vi "record_fiberphotometry_animalbehavior.vi"() -> ()   [LabVIEW 2020]
uses:
  <vilib>/vision/driver/IMAQdx.llb/IMAQdx Buffer Number Mode.ctl
  <vilib>/userDefined/High Color/IMAQdx.ctl
  <userlib>/AndorSDK3/Data/GetPixelData16.vi
  <vilib>/vision/driver/NI_Vision_Acquisition_Software.lvlib
panel:
  in  "Aquisition interval (s)":dbl
  in  "Camera Exposure(s)":dbl
  in  "AOI Top":i64
  in  "AOI Left":i64
  in  "moviefile name":string
  in  "Behavior Data Path":path
  in  "Measurement period (min)":dbl
  in  "Sampling rate (Hz)":i32=5
  in  "error constant":errorcluster
  in  "USB camera":T1
  in  "stop 2":bool
  in  "Buffer Number Mode (Next)":T2
  out "Image":T3(plugin-control)
  in  "405 nm power(%)":i32
  in  "470 nm power (%)":i32
  in  "Imaging Data Path":path
  in  "Binning":string
  in  "Apply Settings":bool
  in  "stop":bool
  in  "count":i32
  in  "image pointers":u64[](array[numeric])
  in  "imageNo":i32 caption="Displayed image" min=0 max=75
  in  "NumImages":i32=10
  in  "Centre AOI":bool
  in  "AOI Width":i64
  in  "AOI Height":i64
  out "Ready":bool
  in  "Run":bool
  in  "error":errorcluster
  out "Pixel Encoding":string
  out "Intensity Graph":u16[][](graph)
  out "AOIStride":i64
  in  "PreAmp Gain Control":string(combo)
  out "PixelData":u16[](array[numeric])
  out "ByteData":u8[](array[numeric])
  out "ImageSizeBytes":i64
  out "Handle":i32
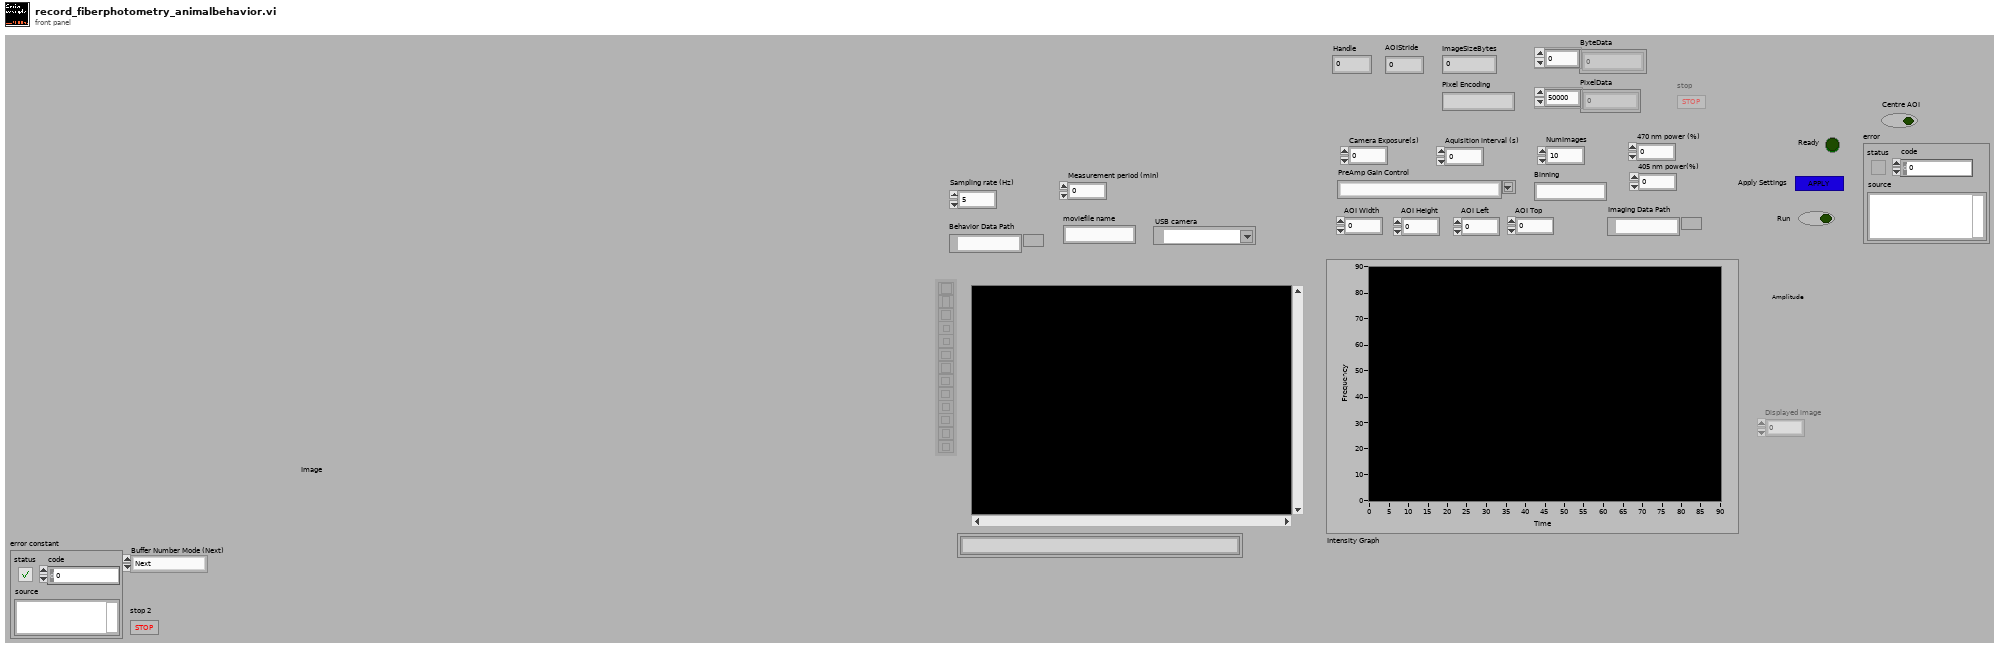
[diagram p1: front panel]
types:
  T1 = typedef "IMAQdx.ctl" = refnum<k21>
  T2 = typedef "NI_Vision_Acquisition_Software.lvlib/IMAQdx Buffer Number Mode.ctl" = enum32{"Next", "Last", "Buffer Number", "Every", "Last New"}
  T3 = typedef "IMAQ Image.ctl" = refnum<image>
  T4 = enum8{"Enabled", "Disabled", "Disabled and Grayed Out"}
  T5 = typedef "Image Type" = u32
  T6 = typedef "AviRefnum.ctl" = refnum<k1>
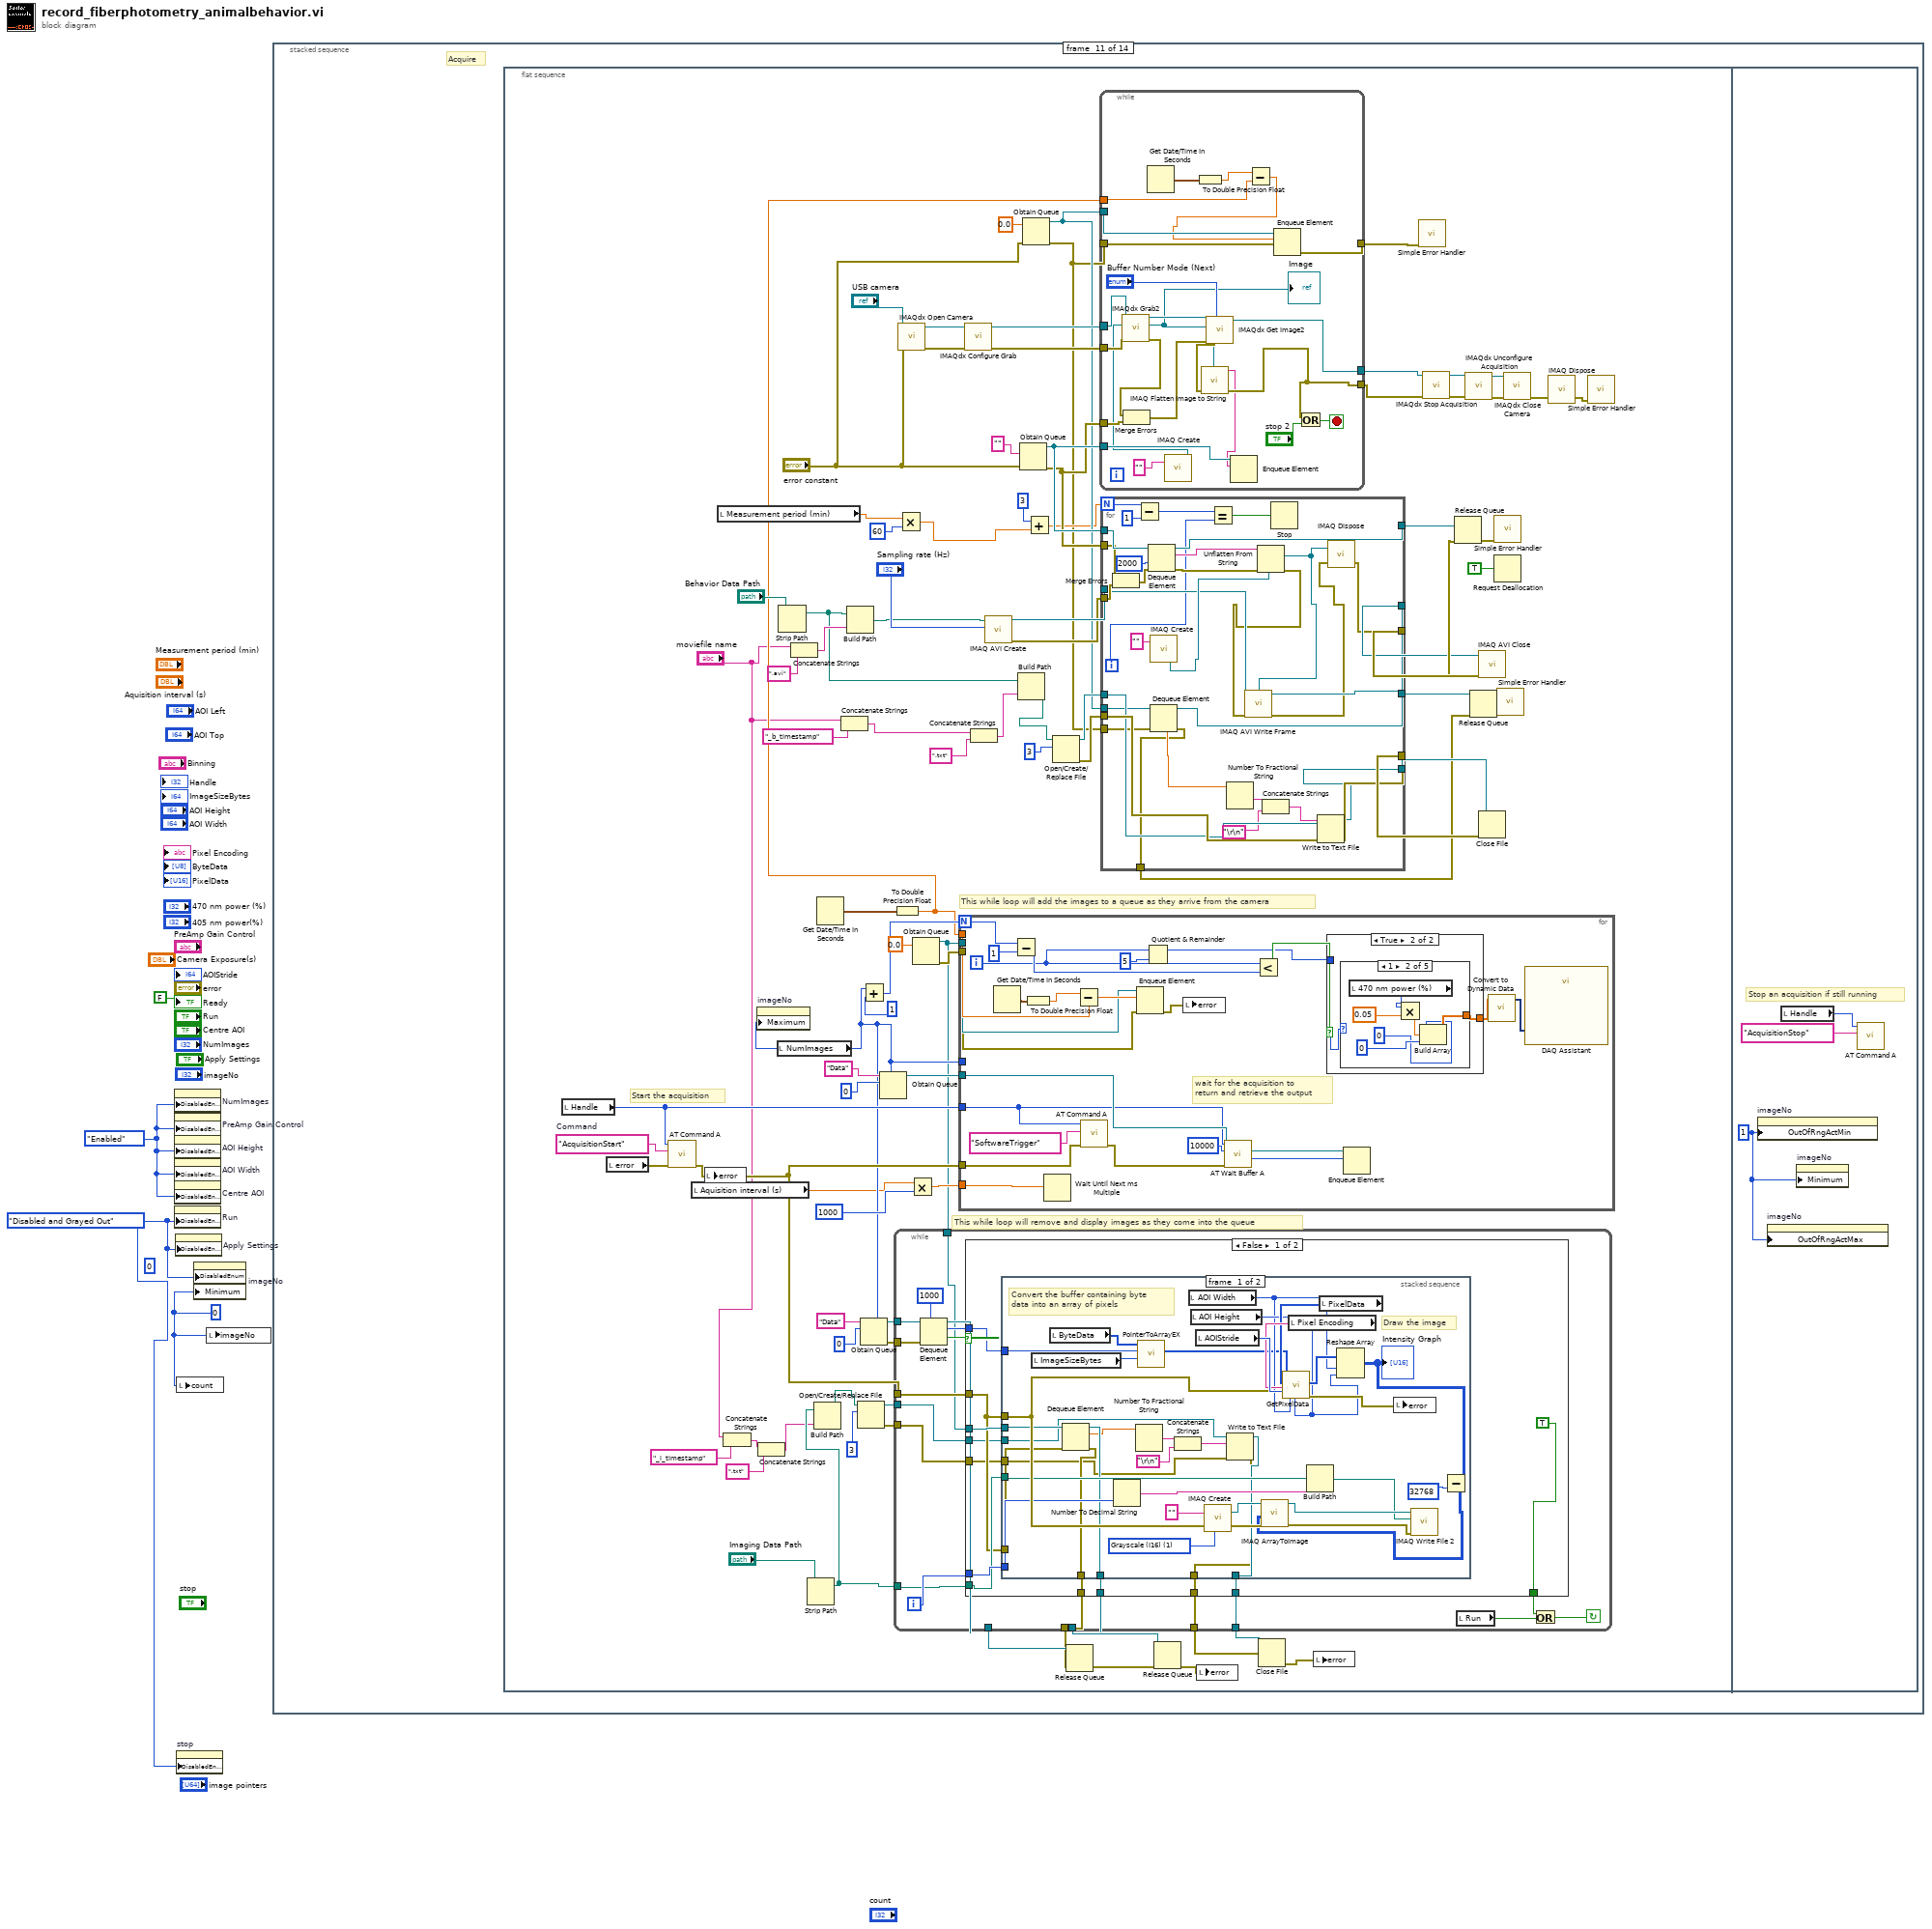
[diagram p0: block diagram]
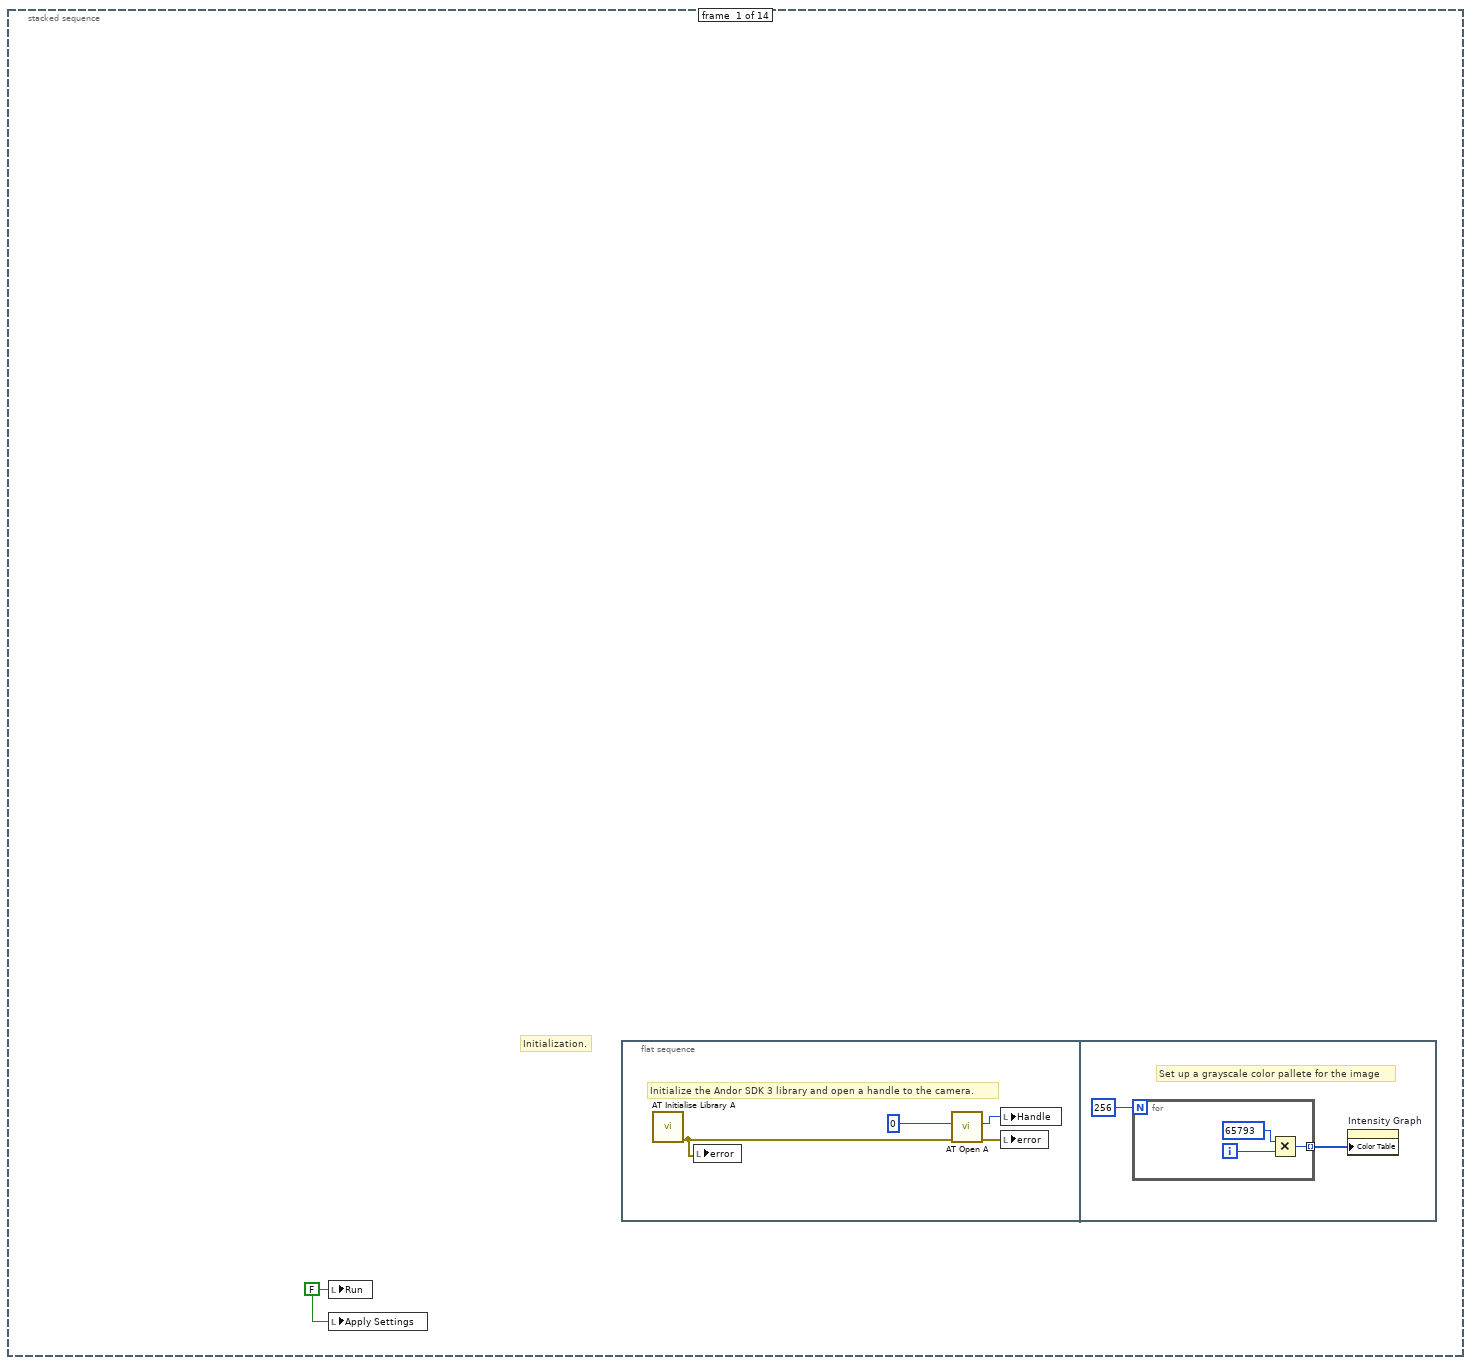
[diagram p2: hidden frame]
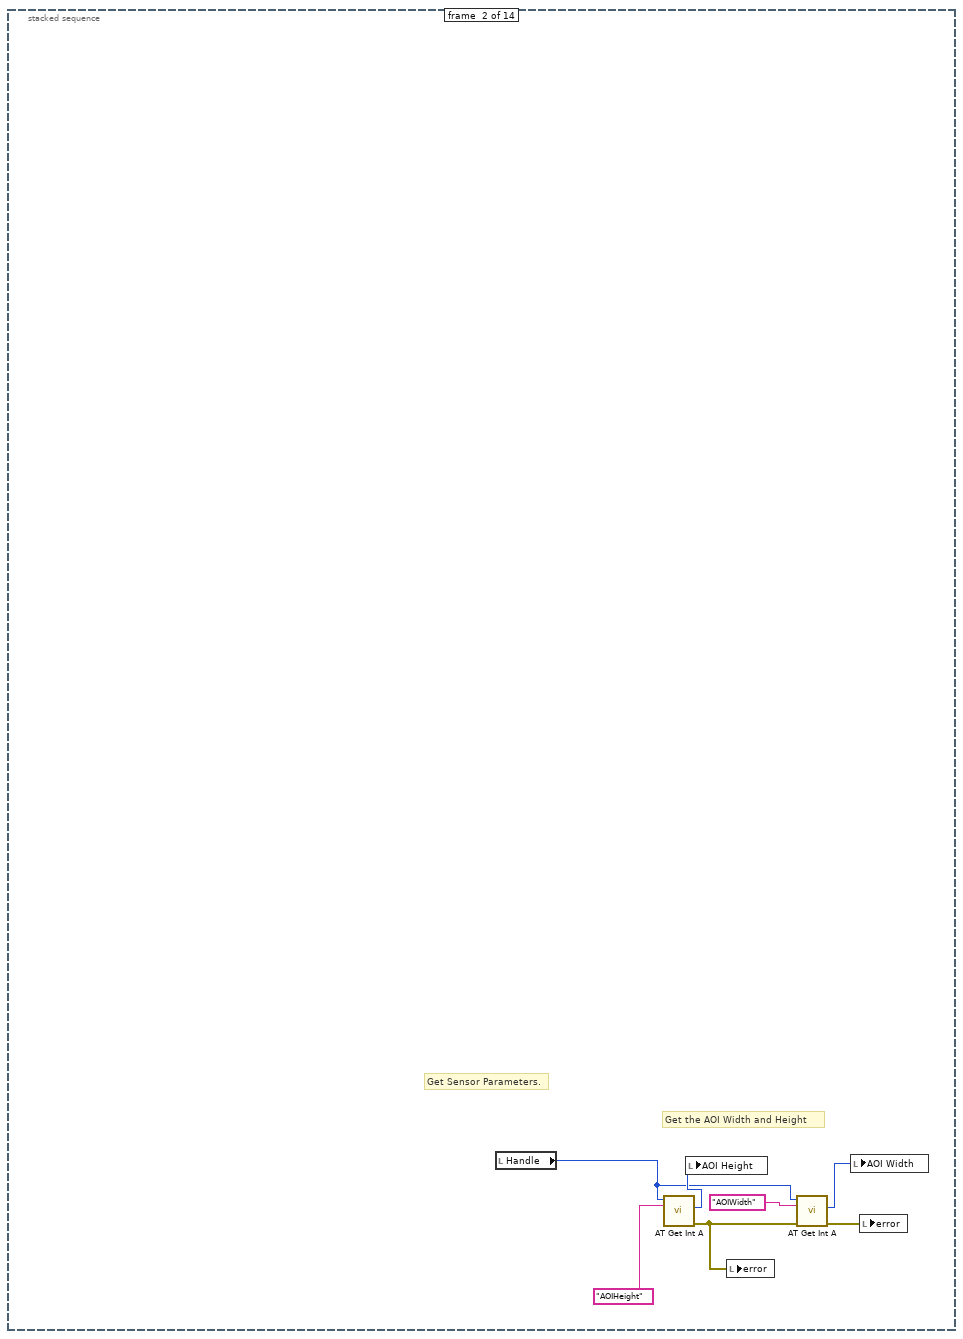
[diagram p3: hidden frame]
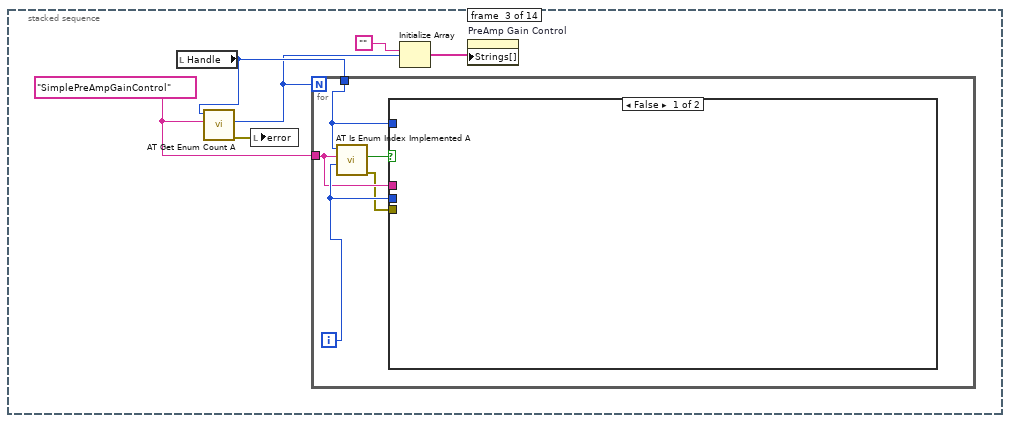
[diagram p4: hidden frame]
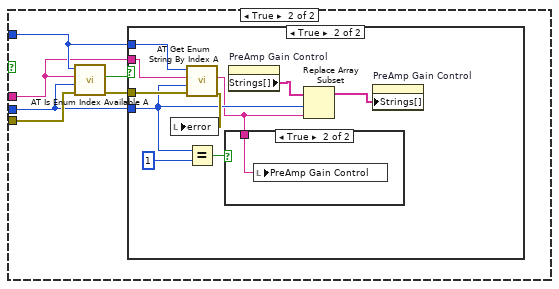
[diagram p5: hidden frame]
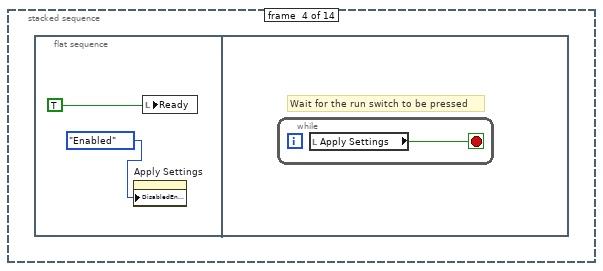
[diagram p8: hidden frame]
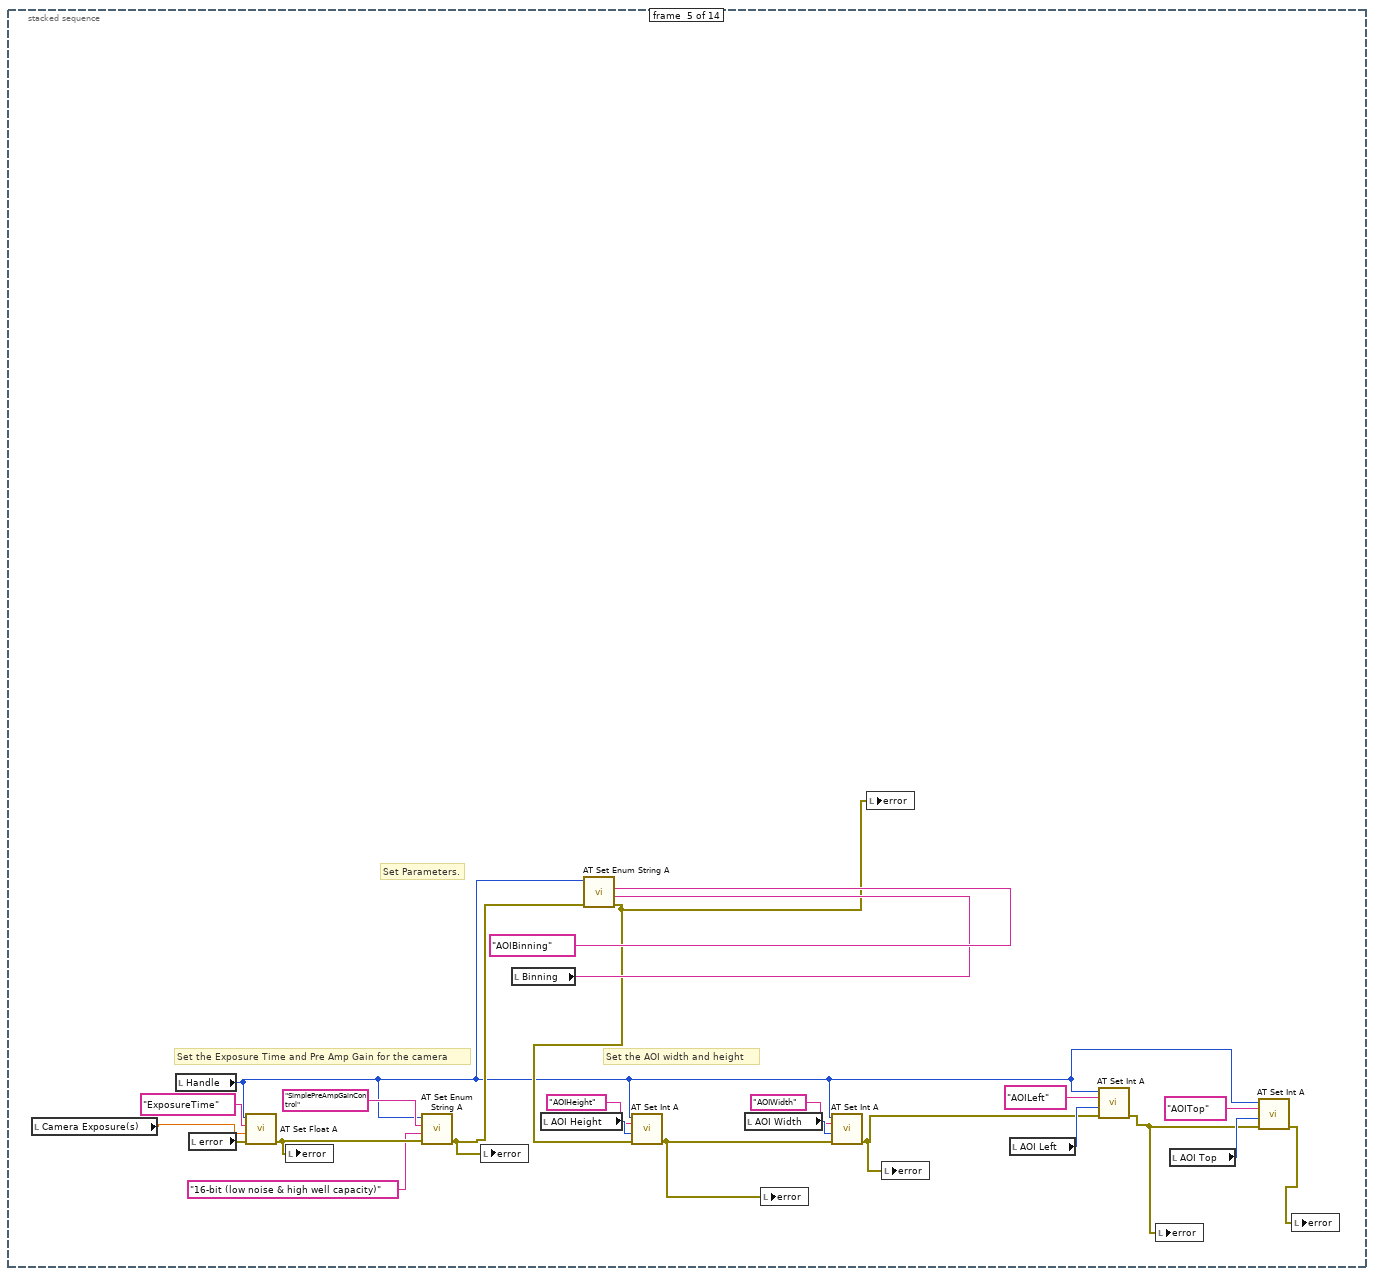
[diagram p9: hidden frame]
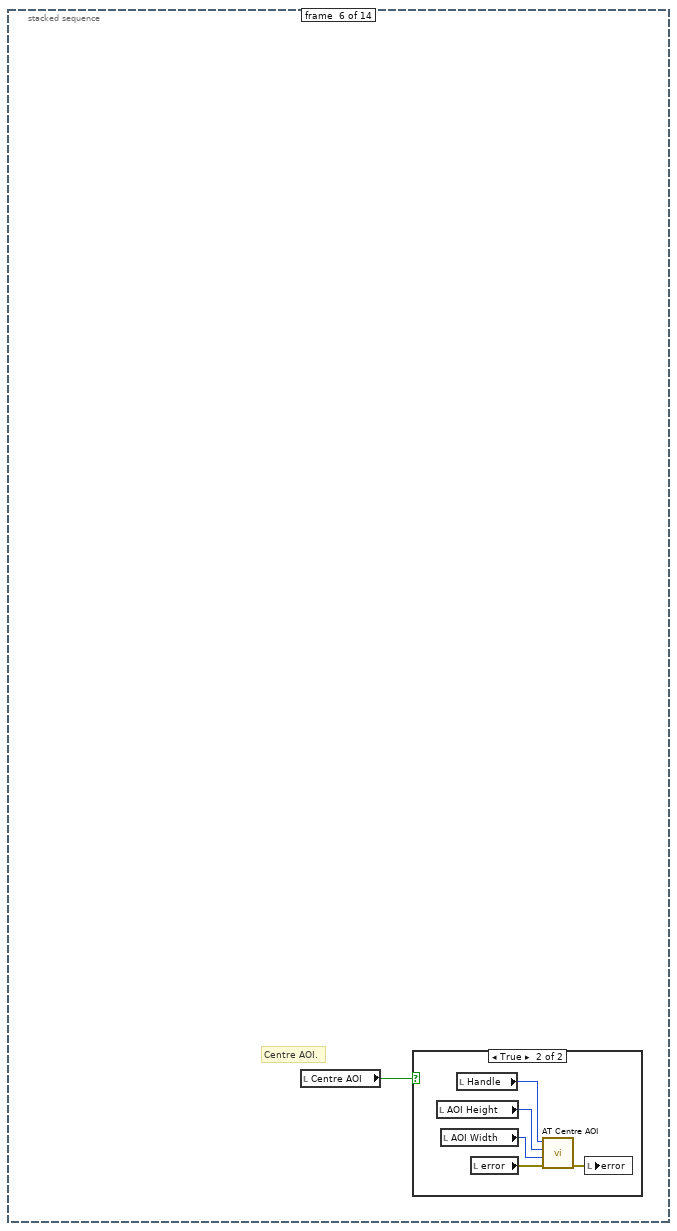
[diagram p10: hidden frame]
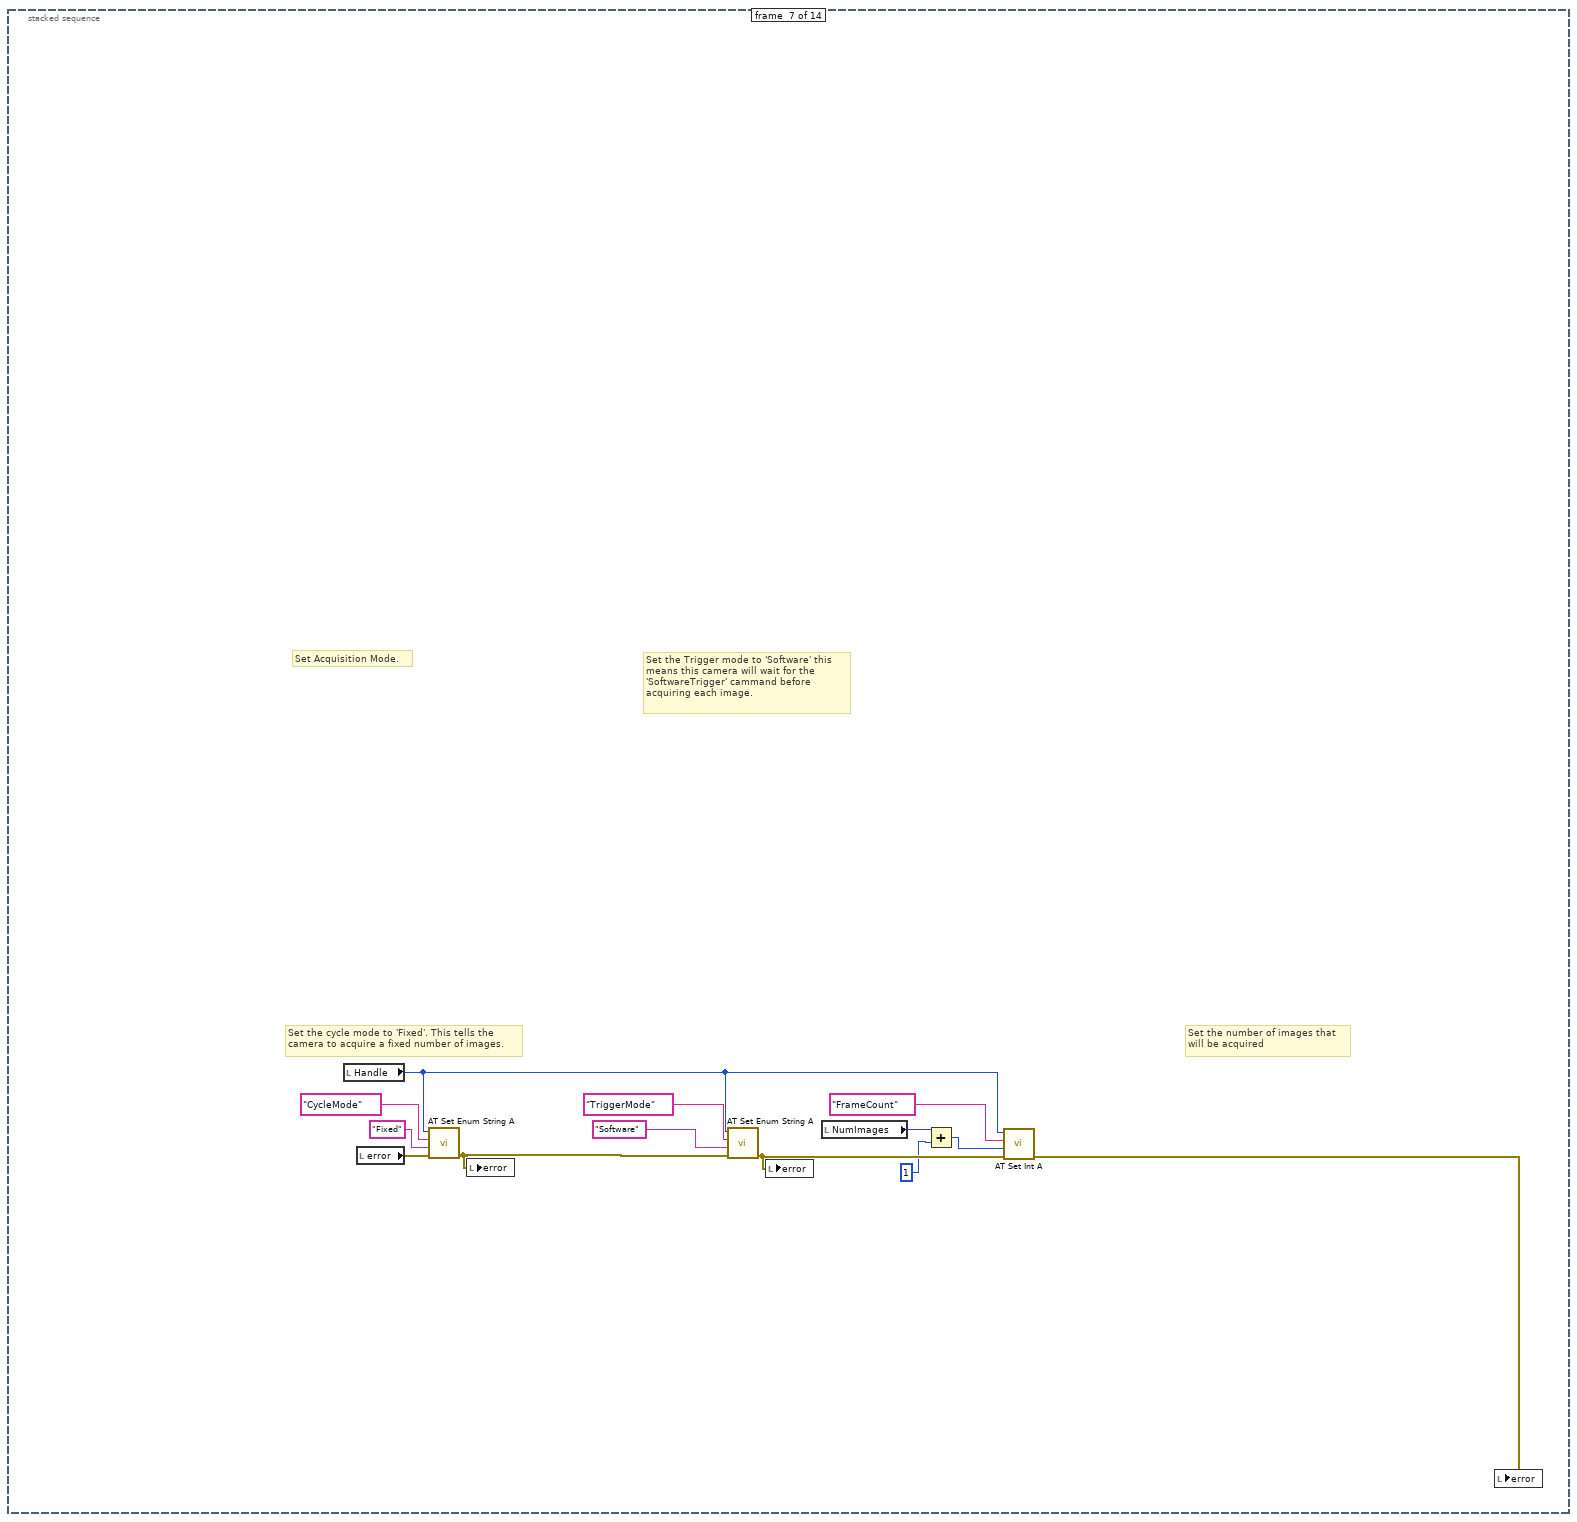
[diagram p12: hidden frame]
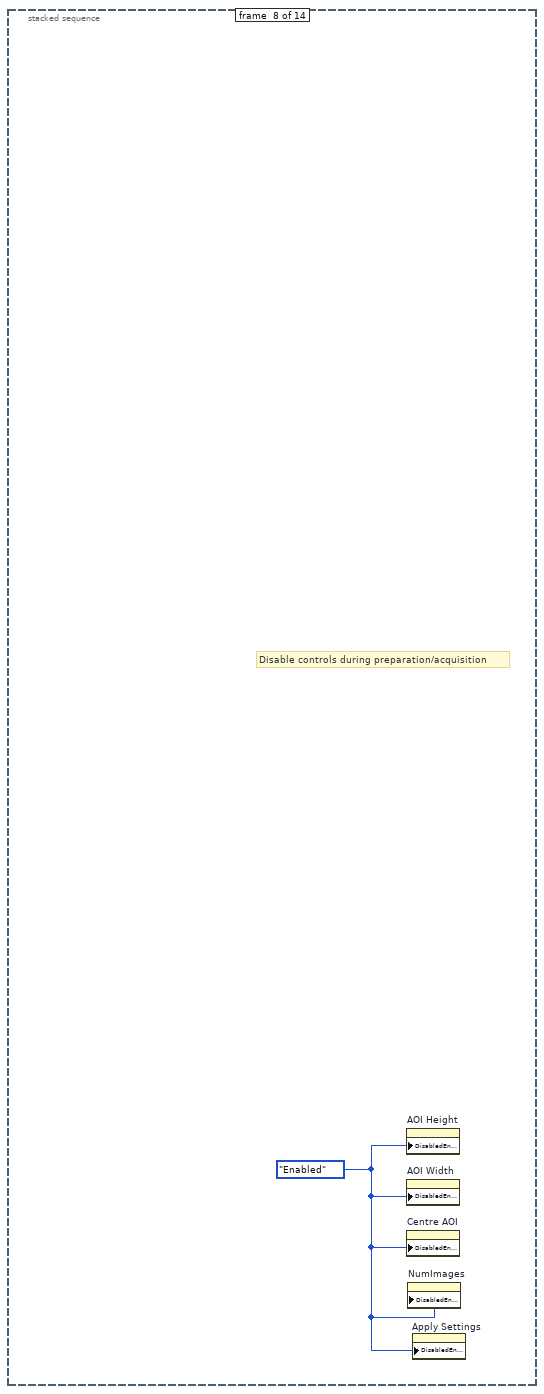
[diagram p13: hidden frame]
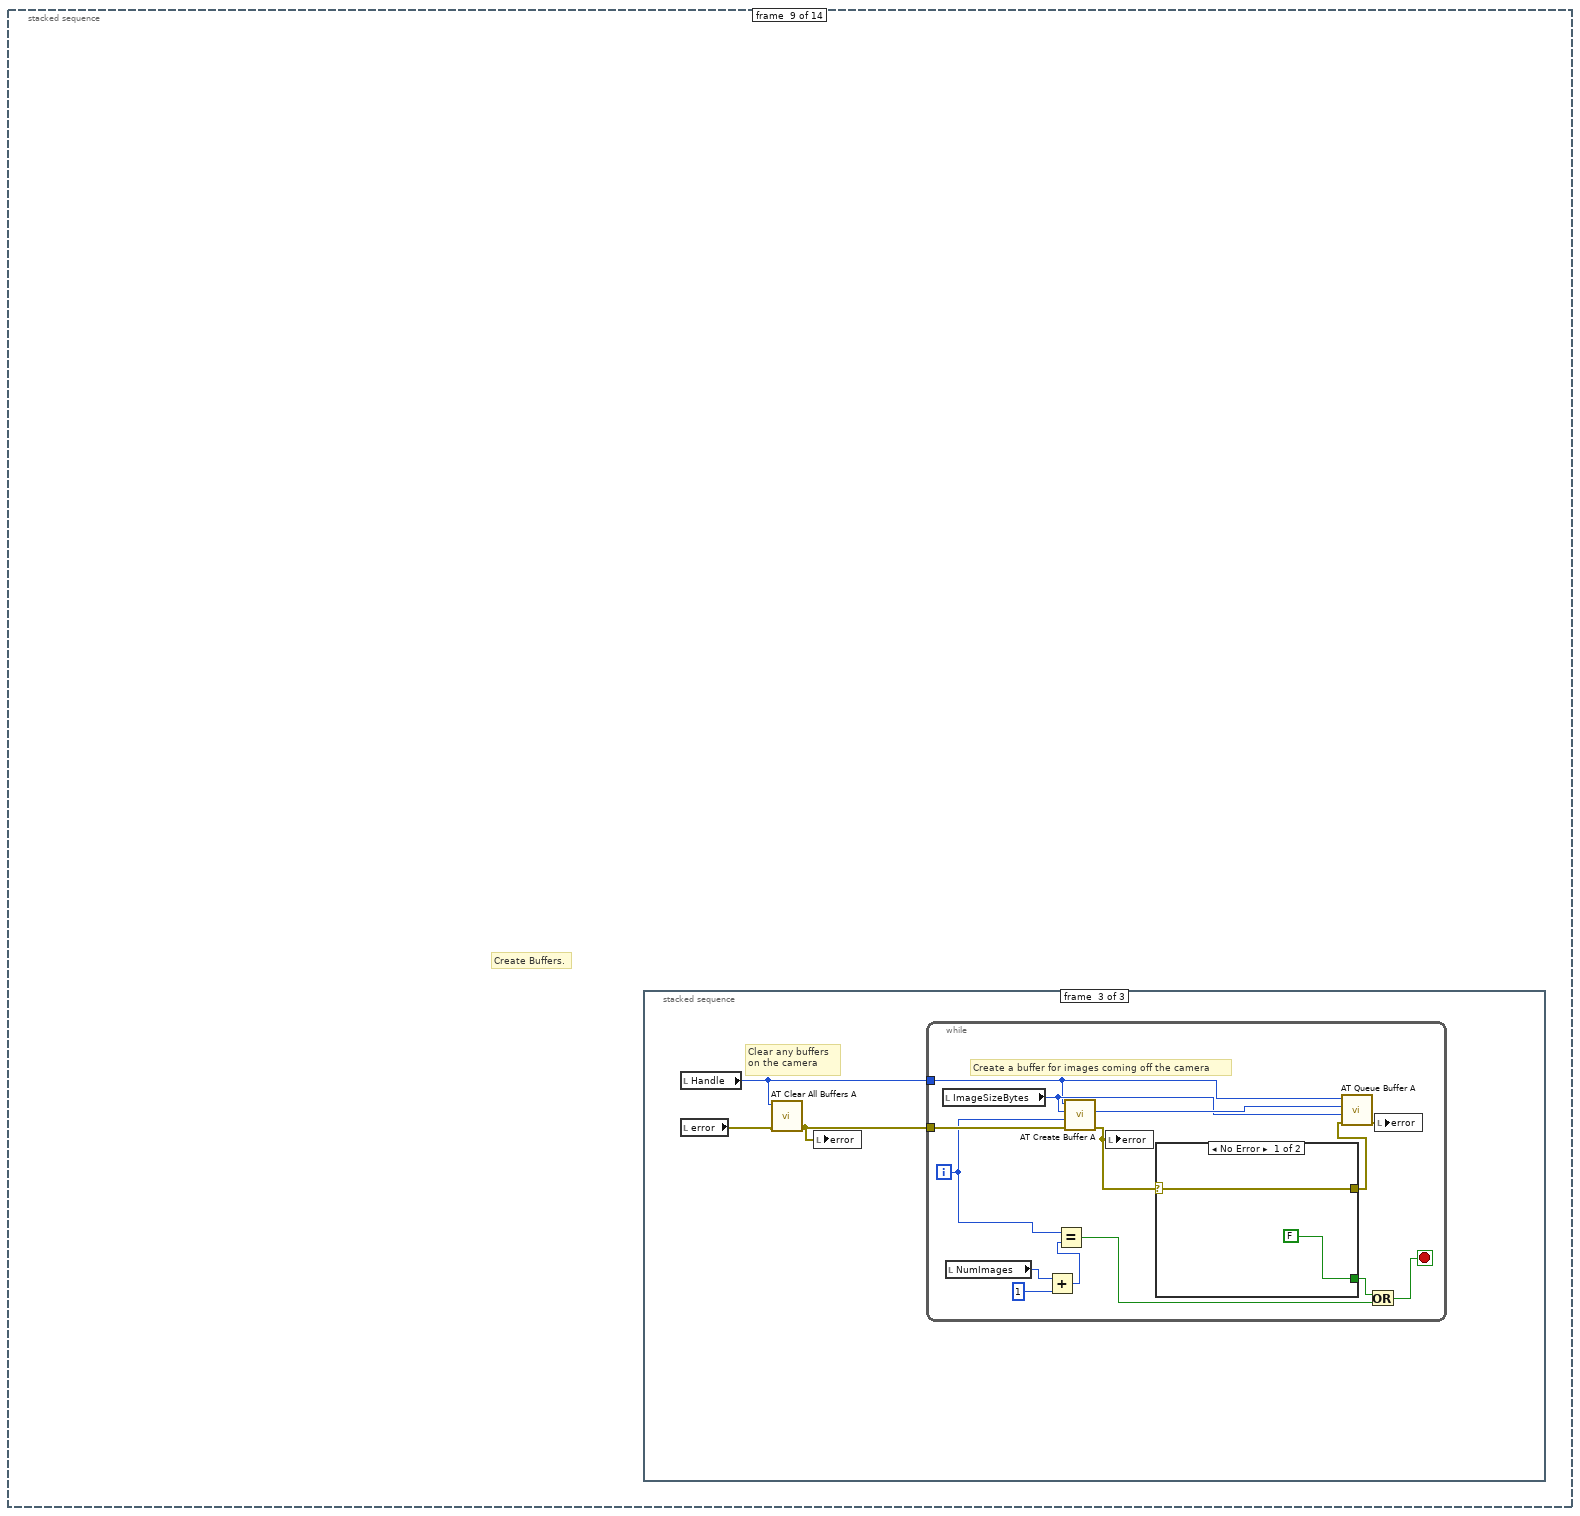
[diagram p14: hidden frame]
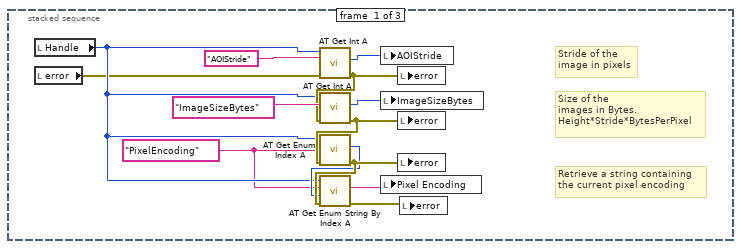
[diagram p15: hidden frame]
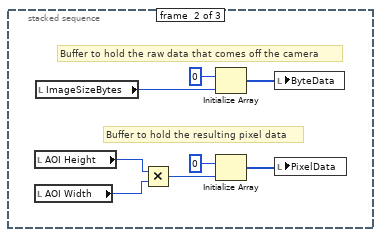
[diagram p16: hidden frame]
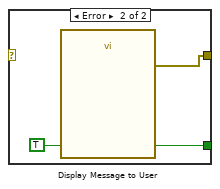
[diagram p17: hidden frame]
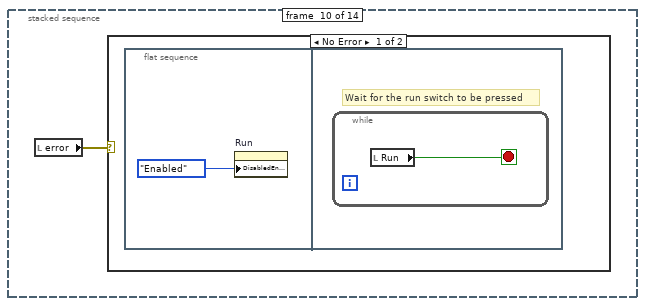
[diagram p18: hidden frame]
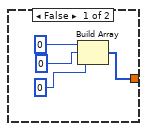
[diagram p20: hidden frame]
diagram:
  w2 = 0 ("Data Entry Limits:Minimum")
  (unwired) 0 ("Image")
  w1 = T4."Disabled and Grayed Out" ("Disabled")
  w3 = T4."Enabled" ("Disabled")
  n1 = property on="NumImages" class="DigNum (strict)"("DisabledEnum"=w3) -> ()  [unwired: 2 in, 2 out]
  n2 = property on="PreAmp Gain Control" class="CmbBox"("DisabledEnum"=w3) -> ()  [unwired: 2 in, 2 out]
  n3 = property on="AOI Height" class="DigNum (strict)"("DisabledEnum"=w3) -> ()  [unwired: 2 in, 2 out]
  n4 = property on="AOI Width" class="DigNum (strict)"("DisabledEnum"=w3) -> ()  [unwired: 2 in, 2 out]
  n5 = property on="Centre AOI" class="Bool (strict)"("DisabledEnum"=w3) -> ()  [unwired: 2 in, 2 out]
  n6 = property on="Run" class="Bool (strict)"("DisabledEnum"=w1) -> ()  [unwired: 2 in, 2 out]
  n7 = property on="Apply Settings" class="Bool (strict)"("DisabledEnum"=w1) -> ()  [unwired: 2 in, 2 out]
  n8 = local write "count"(w2) -> ()
  n9 = property on="stop" class="Bool (strict)"("DisabledEnum"=w1) -> ()  [unwired: 2 in, 2 out]
  n10 = property on="imageNo" class="DigNum (strict)"("DisabledEnum"=w1, "Minimum"=w2) -> ()  [unwired: 2 in, 2 out]
  n11 = local write "imageNo"(w2) -> ()
  n12 = stacked-sequence {
    frame #0 {
      w5 = FALSE ("Run")
      # "Initialization."
      n13 = local write "Run"(w5) -> ()
      n14 = local write "Apply Settings"(w5) -> ()
      n15 = flat-sequence {
        frame #0 {
          # "Initialize the Andor SDK 3 library and open a handle to the camera."
          n16 = call <userlib>:"AT Initialise Library A.vi"() -> ("error out"=w7:errorcluster)  [unwired: 10 in, 1 out]
          n17 = local write "error"(w7) -> ()
          n18 = call <userlib>:"AT Open A.vi"("error in (no error)"=w7, "CameraIndex"=0) -> ("error out"=w6:errorcluster, "Handle"=w8:i32)  [unwired: 7 in, 1 out]
          n19 = local write "Handle"(w8) -> ()
          n20 = local write "error"(w6) -> ()
        }
        frame #1 {
          # "Set up a grayscale color pallete for the image"
          n21 = for {
            N: 256 -> [_]
            tunnel: [w13] -> w10 mode=indexing
            i -> [w14]
            n22 = Multiply(x=65793, y=w14) -> (x*y=w13:i32)
          }
          n23 = property on="Intensity Graph" class="IntGraph (strict)"("Color Table"=w10) -> ()  [unwired: 2 in, 2 out]
        }
      }
    }
    frame #1 {
      # "Get the AOI Width and Height"
      # "Get Sensor Parameters."
      n24 = local read "Handle"() -> (w15:i32)
      n25 = call <userlib>:"AT Get Int A.vi"("Feature"="AOIHeight" ("Integer feature 2"), "Handle"=w15) -> ("error out"=w18:errorcluster, "Value"=w16:i64)  [unwired: 7 in, 1 out]
      n26 = local write "AOI Height"(w16) -> ()
      n27 = local write "error"(w18) -> ()
      n28 = call <userlib>:"AT Get Int A.vi"("error in (no error)"=w18, "Feature"="AOIWidth" ("Integer feature"), "Handle"=w15) -> ("error out"=w21:errorcluster, "Value"=w17:i64)  [unwired: 6 in, 1 out]
      n29 = local write "AOI Width"(w17) -> ()
      n30 = local write "error"(w21) -> ()
    }
    frame #2 {
      w22 = "SimplePreAmpGainControl" ("Enum feature")
      n31 = local read "Handle"() -> (w26:i32)
      n32 = call <userlib>:"AT Get Enum Count A.vi"("Feature"=w22, "Handle"=w26) -> ("error out"=w27:errorcluster, "Count"=w25:i32)  [unwired: 7 in, 1 out]
      n33 = local write "error"(w27) -> ()
      n34 = for {
        N: w25 -> [_]
        tunnel: w26 -> [w29]
        tunnel: w22 -> [w30]
        i -> [w31]
        n35 = call <userlib>:"AT Is Enum Index Implemented A.vi"("Index"=w31, "Feature"=w30, "Handle"=w29) -> ("error out"=w28:errorcluster, "Implemented"=w32:bool)  [unwired: 6 in, 1 out]
        n36 = case shown="False" w32 {
          tunnel: w31 -> [_ w34]
          tunnel: w30 -> [_ w35]
          tunnel: w29 -> [_ w36]
          tunnel: w28 -> [_ w38]
          frame False {
          }
          frame True {
            n37 = call <userlib>:"AT Is Enum Index Available A.vi"("error in (no error)"=w38, "Index"=w34, "Feature"=w35, "Handle"=w36) -> ("error out"=w33:errorcluster, "Available"=w37:bool)  [unwired: 5 in, 1 out]
            n38 = case shown="True" w37 {
              tunnel: w36 -> [_ w48]
              tunnel: w35 -> [_ w47]
              tunnel: w34 -> [_ w44]
              tunnel: w33 -> [_ w46]
              frame False {
              }
              frame True {
                n39 = call <userlib>:"AT Get Enum String By Index A.vi"("error in (no error)"=w46, "Index"=w44, "Feature"=w47, "Handle"=w48) -> ("error out"=w45:errorcluster, "String"=w41:string)  [unwired: 5 in, 1 out]
                n40 = local write "error"(w45) -> ()
                n41 = Equal?(x=w44, y=1) -> (x = y?=w42:bool)
                n42 = case shown="True" w42 {
                  tunnel: w41 -> [_ w49]
                  frame False {
                  }
                  frame True {
                    n43 = local write "PreAmp Gain Control"(w49) -> ()
                  }
                }
                n44 = property on="PreAmp Gain Control" class="CmbBox"() -> ("Strings[]"=w40:string[])  [unwired: 2 in, 2 out]
                n45 = Replace Array Subset(array=w40, new element=w41, index=w44) -> (w39:string[])
                n46 = property on="PreAmp Gain Control" class="CmbBox"("Strings[]"=w39) -> ()  [unwired: 2 in, 2 out]
              }
            }
          }
        }
      }
      n47 = Initialize Array("", w25) -> (w23:string[])
      n48 = property on="PreAmp Gain Control" class="CmbBox"("Strings[]"=w23) -> ()  [unwired: 2 in, 2 out]
    }
    frame #3 {
      n49 = flat-sequence {
        frame #0 {
          n50 = property on="Apply Settings" class="Bool (strict)"("DisabledEnum"=T4."Enabled" ("Disabled")) -> ()  [unwired: 2 in, 2 out]
          n51 = local write "Ready"(TRUE ("Ready")) -> ()
        }
        frame #1 {
          # "Wait for the run switch to be pressed"
          n52 = while {
            stop <- w52 stop-if-true
            n53 = local read "Apply Settings"() -> (w52:bool)
          }
        }
      }
    }
    frame #4 {
      # "Set the AOI width and height"
      # "Set the Exposure Time and Pre Amp Gain for the camera"
      # "Set Parameters."
      n54 = local read "Camera Exposure(s)"() -> (w53:dbl)
      n55 = local read "Handle"() -> (w54:i32)
      n56 = local read "error"() -> (w73:errorcluster)
      n57 = call <userlib>:"AT Set Float A.vi"("error in (no error)"=w73, "Value"=w53, "Feature"="ExposureTime" ("ExposureTime"), "Hndl"=w54) -> ("error out"=w75:errorcluster)  [unwired: 6 in, 1 out]
      n58 = local write "error"(w75) -> ()
      n59 = call <userlib>:"AT Set Enum String A.vi"("error in (no error)"=w75, "String"="16-bit (low noise & high well capacity)", "Feature"="SimplePreAmpGainControl" ("Enum feature"), "Handle"=w54) -> ("error out"=w64:errorcluster)  [unwired: 6 in, 1 out]
      n60 = local write "error"(w64) -> ()
      n61 = local read "Binning"() -> (w65:string)
      n62 = local read "AOI Height"() -> (w71:i64)
      n63 = call <userlib>:"AT Set Enum String A.vi"("error in (no error)"=w64, "String"=w65, "Feature"="AOIBinning" ("Enum feature"), "Handle"=w54) -> ("error out"=w63:errorcluster)  [unwired: 6 in, 1 out]
      n64 = call <userlib>:"AT Set Int A.vi"("error in (no error)"=w63, "Value"=w71, "Feature"="AOIHeight" ("Integer feature"), "Handle"=w54) -> ("error out"=w72:errorcluster)  [unwired: 6 in, 1 out]
      n65 = local read "AOI Width"() -> (w70:i64)
      n66 = local write "error"(w72) -> ()
      n67 = call <userlib>:"AT Set Int A.vi"("error in (no error)"=w72, "Value"=w70, "Feature"="AOIWidth" ("Integer feature 2"), "Handle"=w54) -> ("error out"=w55:errorcluster)  [unwired: 6 in, 1 out]
      n68 = local write "error"(w63) -> ()
      n69 = local write "error"(w55) -> ()
      n70 = local read "AOI Left"() -> (w61:i64)
      n71 = call <userlib>:"AT Set Int A.vi"("error in (no error)"=w55, "Value"=w61, "Feature"="AOILeft" ("Integer feature 2"), "Handle"=w54) -> ("error out"=w56:errorcluster)  [unwired: 6 in, 1 out]
      n72 = local write "error"(w56) -> ()
      n73 = local read "AOI Top"() -> (w59:i64)
      n74 = call <userlib>:"AT Set Int A.vi"("error in (no error)"=w56, "Value"=w59, "Feature"="AOITop" ("Integer feature 2"), "Handle"=w54) -> ("error out"=w57:errorcluster)  [unwired: 6 in, 1 out]
      n75 = local write "error"(w57) -> ()
    }
    frame #5 {
      # "Centre AOI."
      n76 = local read "Centre AOI"() -> (w76:bool)
      n77 = case shown="True" w76 {
        frame False {
        }
        frame True {
          n78 = local read "AOI Height"() -> (w78:i64)
          n79 = local read "AOI Width"() -> (w79:i64)
          n80 = local read "Handle"() -> (w77:i32)
          n81 = local read "error"() -> (w80:errorcluster)
          n82 = call <userlib>:"AT Centre AOI.vi"("error in (no error)"=w80, "AOI Width"=w79, "AOI Height"=w78, "Handle"=w77) -> ("error out"=w81:errorcluster)  [unwired: 7 in]
          n83 = local write "error"(w81) -> ()
        }
      }
    }
    frame #6 {
      # "Set the number of images that \nwill be acquired"
      # "Set the Trigger mode to 'Software' this \nmeans this camera will wait for the \n'SoftwareTrigger' cammand before \nacquiring each image."
      # "Set the cycle mode to 'Fixed'. This tells the \ncamera to acquire a fixed number of images."
      # "Set Acquisition Mode."
      n84 = local read "Handle"() -> (w88:i32)
      n85 = local read "error"() -> (w93:errorcluster)
      n86 = call <userlib>:"AT Set Enum String A.vi"("error in (no error)"=w93, "String"="Fixed", "Feature"="CycleMode" ("Enum feature"), "Handle"=w88) -> ("error out"=w92:errorcluster)  [unwired: 6 in, 1 out]
      n87 = local write "error"(w92) -> ()
      n88 = call <userlib>:"AT Set Enum String A.vi"("error in (no error)"=w92, "String"="Software", "Feature"="TriggerMode" ("Enum feature"), "Handle"=w88) -> ("error out"=w90:errorcluster)  [unwired: 6 in, 1 out]
      n89 = local write "error"(w90) -> ()
      n90 = local read "NumImages"() -> (w84:i32)
      n91 = Add(x=w84, y=1) -> (x+y=w82:i32)
      n92 = call <userlib>:"AT Set Int A.vi"("error in (no error)"=w90, "Value"=w82, "Feature"="FrameCount" ("Integer feature 2"), "Handle"=w88) -> ("error out"=w85:errorcluster)  [unwired: 6 in, 1 out]
      n93 = local write "error"(w85) -> ()
    }
    frame #7 {
      w95 = T4."Enabled" ("Disabled")
      # "Disable controls during preparation/acquisition"
      n94 = property on="AOI Height" class="DigNum (strict)"("DisabledEnum"=w95) -> ()  [unwired: 2 in, 2 out]
      n95 = property on="AOI Width" class="DigNum (strict)"("DisabledEnum"=w95) -> ()  [unwired: 2 in, 2 out]
      n96 = property on="Centre AOI" class="Bool (strict)"("DisabledEnum"=w95) -> ()  [unwired: 2 in, 2 out]
      n97 = property on="NumImages" class="DigNum (strict)"("DisabledEnum"=w95) -> ()  [unwired: 2 in, 2 out]
      n98 = property on="Apply Settings" class="Bool (strict)"("DisabledEnum"=w95) -> ()  [unwired: 2 in, 2 out]
    }
    frame #8 {
      # "Create Buffers."
      n99 = stacked-sequence {
        frame #0 {
          w96 = "PixelEncoding" ("Enum feature")
          # "Retrieve a string containing \nthe current pixel encoding"
          # "Stride of the\nimage in pixels"
          # "Size of the\nimages in Bytes.\nHeight*Stride*BytesPerPixel"
          n100 = local read "Handle"() -> (w98:i32)
          n101 = local read "error"() -> (w97:errorcluster)
          n102 = call <userlib>:"AT Get Int A.vi"("error in (no error)"=w97, "Feature"="AOIStride" ("Integer feature"), "Handle"=w98) -> ("error out"=w104:errorcluster, "Value"=w108:i64)  [unwired: 6 in, 1 out]
          n103 = call <userlib>:"AT Get Int A.vi"("error in (no error)"=w104, "Feature"="ImageSizeBytes" ("Integer feature"), "Handle"=w98) -> ("error out"=w103:errorcluster, "Value"=w107:i64)  [unwired: 6 in, 1 out]
          n104 = call <userlib>:"AT Get Enum Index A.vi"("error in (no error)"=w103, "Feature"=w96, "Handle"=w98) -> ("error out"=w102:errorcluster, "Value"=w101:i32)  [unwired: 6 in, 1 out]
          n105 = call <userlib>:"AT Get Enum String By Index A.vi"("error in (no error)"=w102, "Index"=w101, "Feature"=w96, "Handle"=w98) -> ("error out"=w99:errorcluster, "String"=w100:string)  [unwired: 5 in, 1 out]
          n106 = local write "AOIStride"(w108) -> ()
          n107 = local write "ImageSizeBytes"(w107) -> ()
          n108 = local write "Pixel Encoding"(w100) -> ()
          n109 = local write "error"(w104) -> ()
          n110 = local write "error"(w103) -> ()
          n111 = local write "error"(w102) -> ()
          n112 = local write "error"(w99) -> ()
        }
        frame #1 {
          # "Buffer to hold the resulting pixel data"
          # "Buffer to hold the raw data that comes off the camera"
          n113 = local read "AOI Height"() -> (w114:i64)
          n114 = local read "AOI Width"() -> (w115:i64)
          n115 = local read "ImageSizeBytes"() -> (w110:i64)
          n116 = Multiply(x=w114, y=w115) -> (x*y=w109:i64)
          n117 = Initialize Array(u8 0, w110) -> (w112:u8[])
          n118 = Initialize Array(i64 0, w109) -> (w113:i64[])
          n119 = local write "ByteData"(w112) -> ()
          n120 = local write "PixelData"(w113) -> ()
        }
        frame #2 {
          # "Clear any buffers \non the camera"
          n121 = local read "Handle"() -> (w117:i32)
          n122 = local read "error"() -> (w119:errorcluster)
          n123 = call <userlib>:"AT Clear All Buffers A.vi"("error in (no error)"=w119, "Handle"=w117) -> ("error out"=w118:errorcluster)  [unwired: 8 in, 1 out]
          n124 = local write "error"(w118) -> ()
          n125 = while {
            tunnel: w118 -> [w130]
            tunnel: w117 -> [w129]
            i -> [w126]
            stop <- w123 stop-if-true
            # "Create a buffer for images coming off the camera"
            n126 = local read "ImageSizeBytes"() -> (w132:i64)
            n127 = local read "NumImages"() -> (w122:i32)
            n128 = Add(x=w122, y=1) -> (x+y=w120:i32)
            n129 = Equal?(x=w126, y=w120) -> (x = y?=w124:bool)
            n130 = call <userlib>:"AT Create Buffer A.vi"("error in (no error)"=w130, "Buffer"=w126, "Size"=w132, "Handle"=w129) -> ("error out"=w128:errorcluster, "Buffer out"=w133:u64)  [unwired: 5 in, 1 out]
            n131 = local write "error"(w128) -> ()
            n132 = case shown="No Error" w128 {
              selector: w128 -> [w135 _]
              tunnel: [w135 w137] -> w127
              tunnel: [FALSE ("Enable") w136] -> w125
              frame No Error {
              }
              frame Error {
                w136 = TRUE ("Enable")
                n133 = call "Display Message to User"("Enable"=w136) -> ("error out"=w137:errorcluster)  [unwired: 9 in, 1 out]
              }
            }
            n134 = call <userlib>:"AT Queue Buffer A.vi"("error in (no error)"=w127, "PtrSize"=w132, "Ptr"=w133, "Handle"=w129) -> ("error out"=w131:errorcluster)  [unwired: 6 in, 1 out]
            n135 = Or(x=w125, y=w124) -> (x .or. y?=w123:bool)
            n136 = local write "error"(w131) -> ()
          }
        }
      }
    }
    frame #9 {
      n137 = local read "error"() -> (w138:errorcluster)
      n138 = case shown="No Error" w138 {
        frame No Error {
          n139 = flat-sequence {
            frame #0 {
              n140 = property on="Run" class="Bool (strict)"("DisabledEnum"=T4."Enabled" ("Disabled")) -> ()  [unwired: 2 in, 2 out]
            }
            frame #1 {
              # "Wait for the run switch to be pressed"
              n141 = while {
                stop <- w140 stop-if-true
                n142 = local read "Run"() -> (w140:bool)
              }
            }
          }
        }
        frame Error {
        }
      }
    }
    frame #10 {
      # "Acquire"
      n143 = flat-sequence {
        frame #0 {
          w232 = "AcquisitionStart"  # Command
          # "This while loop will remove and display images as they come into the queue"
          # "This while loop will add the images to a queue as they arrive from the camera"
          # "Start the acquisition"
          n144 = local read "Handle"() -> (w233:i32)
          n145 = local read "error"() -> (w206:errorcluster)
          n146 = call <userlib>:"AT Command A.vi"("error in (no error)"=w206, "Feature"=w232, "Handle"=w233) -> ("error out"=w231:errorcluster)  [unwired: 7 in, 1 out]
          n147 = local read "Aquisition interval (s)"() -> (w144:dbl)
          n148 = local write "error"(w231) -> ()
          n149 = local read "Measurement period (min)"() -> (w141:dbl)
          n150 = Concatenate Strings("moviefile name", "_i_timestamp") -> (w151:string)
          n151 = Concatenate Strings(w151, ".txt" ("string")) -> (w150:string)
          n152 = local read "NumImages"() -> (w218:i32)
          n153 = property on="imageNo" class="DigNum (strict)"("Maximum"=w218) -> ()  [unwired: 2 in, 2 out]
          n154 = Strip Path(path="Behavior Data Path") -> (stripped path=w157:path)  [unwired: 1 out]
          n155 = Concatenate Strings("moviefile name", ".avi" ("string")) -> (w159:string)
          n156 = Strip Path(path="Imaging Data Path") -> (stripped path=w154:path)  [unwired: 1 out]
          n157 = Build Path(base path=w154, name or relative path=w150) -> (appended path=w148:path)
          n158 = Get Date/Time In Seconds() -> (seconds since 1Jan1904=w215:timestamp)
          n159 = Concatenate Strings("moviefile name", "_b_timestamp") -> (w155:string)
          n160 = Build Path(base path=w157, name or relative path=w159) -> (appended path=w158:path)
          n161 = Open/Create/Replace File(file path (use dialog)=w148, operation (0:open)=3 ("timeout in ms (-1)")) -> (refnum out=w146:refnum<file>, error out=w147:errorcluster)  [unwired: 4 in, 1 out]
          n162 = Obtain Queue(max queue size (-1, unlimited)=w218, name (unnamed)="Data", element data type=u64 0) -> (queue out=w226:refnum<queue>, error out=w227:errorcluster)  [unwired: 2 in, 1 out]
          n163 = Add(x=w218, y=1) -> (x+y=w217:i32)
          n164 = Obtain Queue(max queue size (-1, unlimited)=w218, name (unnamed)="Data", element data type=u64 0) -> (queue out=w229:refnum<queue>)  [unwired: 2 in, 2 out]
          n165 = To Double Precision Float(number=w215) -> (double precision float=w143:dbl)
          n166 = Multiply(x=w141, y=60 ("timeout in ms (-1)")) -> (x*y=w145:dbl)
          n167 = call <vilib>:"IMAQdx Open Camera.vi"("error in"="error constant", "Session In"="USB camera") -> ("error out"=w203:errorcluster, "Session Out"=w204:T1)  [unwired: 8 in]
          n168 = Multiply(x=w144, y=1000) -> (x*y=w221:dbl)
          n169 = Obtain Queue(element data type=0.0) -> (queue out=w213:refnum<queue>, error out=w214:errorcluster)  [unwired: 4 in, 1 out]
          n170 = while {
            tunnel: w227 -> [w368]
            tunnel: w226 -> [w367]
            tunnel: w231 -> [w366]
            tunnel: [w362] -> w223
            tunnel: w154 -> [w357]
            tunnel: w213 -> [w356]
            tunnel: [w355] -> w212
            tunnel: [w354] -> w211
            tunnel: [w353] -> w209
            tunnel: [w352] -> w208
            tunnel: w147 -> [w351]
            tunnel: w146 -> [w350]
            i -> [w358]
            stop <- w361 continue-if-true
            n171 = Dequeue Element(queue=w367, timeout in ms (-1)=1000, error in (no error)=w368) -> (queue out=w362:refnum<queue>, element=w364:u64, timed out?=w363:bool)  [unwired: 1 out]
            n172 = case shown="False" w363 {
              tunnel: w366 -> [w374 _]
              tunnel: w364 -> [w380 _]
              tunnel: [TRUE ("x") FALSE ("x")] -> w359
              tunnel: w358 -> [w378 _]
              tunnel: w357 -> [w377 _]
              tunnel: w356 -> [w376 _]
              tunnel: [w375 _] -> w355
              tunnel: [w373 _] -> w354
              tunnel: [w372 _] -> w353
              tunnel: [w371 _] -> w352
              tunnel: w351 -> [w370 _]
              tunnel: w350 -> [w369 _]
              frame False {
                n173 = stacked-sequence {
                  tunnel: w374 -> [w403 _]
                  tunnel: w380 -> [w408 w422]
                  tunnel: w378 -> [w399 _]
                  tunnel: w377 -> [w398 _]
                  tunnel: w376 -> [w392 _]
                  tunnel: [w391 _] -> w375
                  tunnel: w374 -> [w386 _]
                  tunnel: [w384 _] -> w373
                  tunnel: [w385 _] -> w372
                  tunnel: [w383 _] -> w371
                  tunnel: w370 -> [w382 _]
                  tunnel: w369 -> [w381 _]
                  frame #0 {
                    w406 = T5 1 items=["Grayscale (U8)", "Grayscale (I16)", "Grayscale (SGL)", "Complex (CSG)", "RGB (U32)", "HSL (U32)", "RGB (U64)"] ("Image Type")
                    # "Draw the image"
                    # "Convert the buffer containing byte \ndata into an array of pixels"
                    n174 = local read "ImageSizeBytes"() -> (w409:i64)
                    n175 = local read "ByteData"() -> (w407:u8[])
                    n176 = Dequeue Element(queue=w392, error in (no error)=w386) -> (queue out=w391:refnum<queue>, element=w390:dbl, error out=w384:errorcluster)  [unwired: 1 in, 1 out]
                    n177 = Number To Decimal String(number=w399) -> (decimal integer string=w400:string)  [unwired: 1 in]
                    n178 = Number To Fractional String(number=w390) -> (F-format string=w389:string)  [unwired: 3 in]
                    n179 = call <userlib>:"PointerToArrayEX.vi"("Array in"=w407, "Pointer In"=w408, "Pointer Size"=w409) -> ("Array out"=w410:u8[])  [unwired: 5 in, 1 out]
                    n180 = Concatenate Strings(w389, "\r\n") -> (w387:string)
                    n181 = local read "AOI Width"() -> (w411:i64)
                    n182 = local read "AOI Height"() -> (w412:i64)
                    n183 = local read "AOIStride"() -> (w417:i64)
                    n184 = call "IMAQ Create"("Image Name"="", "Image Type"=w406, "error in (no error)"=w403) -> ("New Image"=w404:T3, "error out"=w402:errorcluster)  [unwired: 1 in, 1 out]
                    n185 = Write to Text File(file (use dialog)=w381, text=w387, error in=w382) -> (refnum out=w385:refnum<file>, error out=w383:errorcluster)  [unwired: 1 in, 1 out]
                    n186 = local read "Pixel Encoding"() -> (w416:string)
                    n187 = Build Path(base path=w398, name or relative path=w400) -> (appended path=w396:path)
                    n188 = local read "PixelData"() -> (w415:u16[])
                    n189 = call-poly <userlib>:"GetPixelData.vi"("Input buffer"=w410, "Output buffer in"=w415, "Pixel Encoding"=w416, "Stride"=w417, "error in (no error)"=w403, "Width"=w411, "Height"=w412) -> ("Output buffer out"=w413:u16[], "error out"=w414:errorcluster)  [unwired: 10 in, 1 out]
                    n190 = Reshape Array(w413, w411, w412) -> (w393:u16[][])
                    "Intensity Graph" <- w393
                    n191 = local write "error"(w414) -> ()
                    n192 = Subtract(x=w393, y=u64 32768 ("element data type")) -> (x-y=w394:u64[][])
                    n193 = call "IMAQ ArrayToImage"("error in (no error)"=w402, "Image Pixels (I16)"=w394, "Image"=w404) -> ("error out"=w401:errorcluster, "Image Out"=w397:T3)  [unwired: 3 in, 4 out]
                    n194 = call-poly "IMAQ Write File 2"("error in (no error)"=w401, "File Path"=w396, "Image"=w397) -> ()  [unwired: 7 in, 2 out]
                  }
                  frame #1 {
                    # "Store the pointer to the image so we can display\nin order after the acquisition finishes"
                    n195 = local read "image pointers"() -> (w421:u64[])
                    n196 = local read "imageNo"() -> (w418:i32)
                    n197 = Insert Into Array(array=w421, index=w418, new element=w422) -> (w420:u64[])
                    n198 = Increment(x=w418) -> (x+1=w419:i32)
                    n199 = local write "image pointers"(w420) -> ()
                    n200 = local write "imageNo"(w419) -> ()
                  }
                }
              }
              frame True {
              }
            }
            n201 = local read "Run"() -> (w360:bool)
            n202 = Or(x=w359, y=w360) -> (x .or. y?=w361:bool)
          }
          n203 = for {
            N: w217 -> [w306]
            tunnel: w233 -> [w312]
            tunnel: w231 -> [w310]
            tunnel: w229 -> [w314]
            tunnel: w218 -> [_]
            tunnel: w221 -> [w308]
            tunnel: w143 -> [w297]
            tunnel: w213 -> [w295]
            tunnel: w214 -> [w294]
            i -> [w300]
            # "wait for the acquisition to \nreturn and retrieve the output"
            n204 = Get Date/Time In Seconds() -> (seconds since 1Jan1904=w298:timestamp)
            n205 = Subtract(x=w306, y=1) -> (x-y=w301:i32)
            n206 = To Double Precision Float(number=w298) -> (double precision float=w299:dbl)
            n207 = Wait Until Next ms Multiple(millisecond multiple=w308) -> ()  [unwired: 1 out]
            n208 = Subtract(x=w299, y=w297) -> (x-y=w296:dbl)
            n209 = call <userlib>:"AT Command A.vi"("error in (no error)"=w310, "Feature"="SoftwareTrigger" ("Command"), "Handle"=w312) -> ("error out"=w309:errorcluster)  [unwired: 7 in, 1 out]
            n210 = Enqueue Element(queue=w295, element=w296, error in (no error)=w294) -> (error out=w293:errorcluster)  [unwired: 1 in, 2 out]
            n211 = Quotient & Remainder(x=w300, y=5) -> (x-y*floor(x/y)=w302:i32)  [unwired: 1 out]
            n212 = local write "error"(w293) -> ()
            n213 = call <userlib>:"AT Wait Buffer A.vi"("error in (no error)"=w309, "Timeout"=u32 10000, "Handle"=w312) -> ("Output buffer"=w313:u64)  [unwired: 5 in, 3 out]
            n214 = Less?(x=w300, y=w301) -> (x < y?=w303:bool)
            n215 = case shown="True" w303 {
              tunnel: [w317 w321] -> w304
              tunnel: w302 -> [_ w320]
              frame False {
                n216 = Build Array(0, 0, 0) -> (w317:i32[])
              }
              frame True {
                n217 = case shown="1" w320 {
                  tunnel: [w327 w333 w339 w345 w349] -> w321
                  frame 0, Default {
                    n218 = local read "470 nm power (%)"() -> (w324:i32)
                    n219 = Multiply(x=w324, y=0.05) -> (x*y=w322:dbl)
                    n220 = Build Array(0, w322, 0) -> (w327:dbl[])
                  }
                  frame 1 {
                    n221 = local read "470 nm power (%)"() -> (w328:i32)
                    n222 = Multiply(x=w328, y=0.05) -> (x*y=w330:dbl)
                    n223 = Build Array(0, w330, 0) -> (w333:dbl[])
                  }
                  frame 2 {
                    n224 = local read "405 nm power(%)"() -> (w334:i32)
                    n225 = Multiply(x=w334, y=0.05) -> (x*y=w335:dbl)
                    n226 = Build Array(w335, 0, 0) -> (w339:dbl[])
                  }
                  frame 3 {
                    n227 = local read "405 nm power(%)"() -> (w340:i32)
                    n228 = Multiply(x=w340, y=0.05) -> (x*y=w341:dbl)
                    n229 = Build Array(w341, 0, 0) -> (w345:dbl[])
                  }
                  frame 4 {
                    n230 = Build Array(0, 0, 0) -> (w349:i32[])
                  }
                }
              }
            }
            n231 = Enqueue Element(queue=w314, element=w313) -> ()  [unwired: 2 in, 3 out]
            n232 = call "Convert to Dynamic Data"("Array"=w304) -> ("Dynamic Data Type"=w292:dynamicdata)  [unwired: 3 in]
            n233 = call "DAQ Assistant"("data"=w292) -> ()  [unwired: 17 in, 2 out]
          }
          n234 = call <vilib>:"IMAQdx Configure Grab.vi"("error in"=w203, "Session In"=w204) -> ("error out"=w191:errorcluster, "Session Out"=w193:T1)  [unwired: 8 in]
          n235 = Concatenate Strings(w155, ".txt" ("string")) -> (w181:string)
          n236 = call "IMAQ AVI Create"("Frames Per Second"="Sampling rate (Hz)", "AVI Path"=w158) -> ("error out"=w187:errorcluster, "Avi Refnum"=w188:T6)  [unwired: 5 in, 3 out]
          n237 = Build Path(base path=w157, name or relative path=w181) -> (appended path=w180:path)
          n238 = Obtain Queue(element data type="", error in (no error)="error constant") -> (queue out=w195:refnum<queue>, error out=w194:errorcluster)  [unwired: 3 in, 1 out]
          n239 = Obtain Queue(element data type=0.0, error in (no error)="error constant") -> (queue out=w169:refnum<queue>, error out=w163:errorcluster)  [unwired: 3 in, 1 out]
          n240 = Add(x=3 ("timeout in ms (-1)"), y=w145) -> (x+y=w165:dbl)
          n241 = Open/Create/Replace File(file path (use dialog)=w180, operation (0:open)=3 ("timeout in ms (-1)")) -> (refnum out=w178:refnum<file>, error out=w179:errorcluster)  [unwired: 4 in, 1 out]
          n242 = Release Queue(queue=w223) -> ()  [unwired: 2 in, 3 out]
          n243 = while {
            tunnel: [w280] -> w196
            tunnel: w195 -> [w290]
            tunnel: w194 -> [w289]
            tunnel: w193 -> [w282]
            tunnel: [w283] -> w192
            tunnel: w191 -> [w287]
            tunnel: w143 -> [w272]
            tunnel: w169 -> [w270]
            tunnel: w163 -> [w268]
            tunnel: [w267] -> w170
            stop <- w274 stop-if-true
            n244 = Get Date/Time In Seconds() -> (seconds since 1Jan1904=w273:timestamp)
            n245 = call "IMAQ Create"("Image Name"="") -> ("New Image"=w281:T3)  [unwired: 4 in, 1 out]
            n246 = call <vilib>:"IMAQdx Grab2.vi"("error in"=w287, "Image In"=w281, "Session In"=w282) -> ("error out"=w286:errorcluster, "Image Out"=w275:T3, "Session Out"=w288:T1)  [unwired: 5 in, 1 out]
            "Image" <- w275
            n247 = Merge Errors(w286, w289) -> (w285:errorcluster)
            n248 = To Double Precision Float(number=w273) -> (double precision float=w271:dbl)
            n249 = call <vilib>:"IMAQdx Get Image2.vi"("Buffer Number Mode (Next)"="Buffer Number Mode (Next)", "error in"=w285, "Image In"=w275, "Session In"=w288) -> ("error out"=w278:errorcluster, "Image Out"=w276:T3, "Session Out"=w283:T1)  [unwired: 4 in, 1 out]
            n250 = call "IMAQ Flatten Image to String"("error in (no error)"=w278, "Image"=w276) -> ("error out"=w280:errorcluster, "Data String"=w279:string)  [unwired: 8 in]
            n251 = Enqueue Element(queue=w290, element=w279) -> ()  [unwired: 2 in, 3 out]
            n252 = Subtract(x=w271, y=w272) -> (x-y=w269:dbl)
            n253 = Enqueue Element(queue=w270, element=w269, error in (no error)=w268) -> (error out=w267:errorcluster)  [unwired: 1 in, 2 out]
            n254 = Or(x=w280, y="stop 2") -> (x .or. y?=w274:bool)
          }
          n255 = for {
            N: w165 -> [w248]
            tunnel: w195 -> [w266]
            tunnel: w194 -> [w260]
            tunnel: [w265] -> w189
            tunnel: [w240] -> w186
            tunnel: w187 -> [w258]
            tunnel: w188 -> [w257]
            tunnel: [w255] -> w184
            tunnel: w179 -> [w254]
            tunnel: w178 -> [w253]
            tunnel: [w252] -> w177
            tunnel: [w251] -> w176
            tunnel: w169 -> [w245]
            tunnel: [w243] -> w167
            tunnel: w163 -> [w238]
            tunnel: [w237] -> w162
            i -> [w239]
            n256 = Merge Errors(w260, w258) -> (w259:errorcluster)
            n257 = Subtract(x=w248, y=1 ("timeout in ms (-1)")) -> (x-y=w247:i32)
            n258 = Dequeue Element(queue=w266, timeout in ms (-1)=2000, error in (no error)=w259) -> (queue out=w265:refnum<queue>, element=w263:string, error out=w262:errorcluster)  [unwired: 1 out]
            n259 = call "IMAQ Create"("Image Name"="") -> ("New Image"=w261:T3)  [unwired: 3 in, 2 out]
            n260 = Dequeue Element(queue=w245, error in (no error)=w238) -> (queue out=w243:refnum<queue>, element=w244:dbl, error out=w237:errorcluster)  [unwired: 1 in, 1 out]
            n261 = Equal?(x=w247, y=w239) -> (x = y?=w249:bool)
            n262 = Number To Fractional String(number=w244) -> (F-format string=w235:string)  [unwired: 3 in]
            n263 = Unflatten From String(type=w261, binary string=w263, error in (no error)=w262) -> (value=w250:T3, error out=w256:errorcluster)  [unwired: 2 in, 1 out]
            n264 = call "IMAQ AVI Write Frame"("error in (no error)"=w256, "Image"=w250, "Avi Refnum"=w257) -> ("error out"=w241:errorcluster, "Avi Refnum (duplicate)"=w255:T6)  [unwired: 1 in, 6 out]
            n265 = Concatenate Strings(w235, "\r\n") -> (w234:string)
            n266 = Stop(stop? (T)=w249) -> ()
            n267 = Write to Text File(file (use dialog)=w253, text=w234, error in=w254) -> (refnum out=w251:refnum<file>, error out=w252:errorcluster)  [unwired: 1 in, 1 out]
            n268 = call "IMAQ Dispose"("Image"=w250, "error in (no error)"=w241) -> ("error out"=w240:errorcluster)  [unwired: 4 in]
          }
          n269 = Release Queue(queue=w212, error in (no error)=w211) -> (error out=w210:errorcluster)  [unwired: 1 in, 2 out]
          n270 = local write "error"(w210) -> ()
          n271 = Close File(refnum=w209, error in=w208) -> (error out=w207:errorcluster)  [unwired: 1 out]
          n272 = local write "error"(w207) -> ()
          n273 = call <vilib>:"Simple Error Handler.vi"("error in (no error)"=w170) -> ()  [unwired: 4 in, 5 out]
          n274 = call <vilib>:"IMAQdx Stop Acquisition.vi"("error in"=w196, "Session In"=w192) -> ("error out"=w202:errorcluster, "Session Out"=w201:T1)  [unwired: 8 in]
          n275 = call <vilib>:"IMAQdx Unconfigure Acquisition.vi"("error in"=w202, "Session In"=w201) -> ("error out"=w200:errorcluster, "Session Out"=w199:T1)  [unwired: 8 in]
          n276 = Release Queue(queue=w167, error in (no error)=w162) -> (error out=w168:errorcluster)  [unwired: 1 in, 2 out]
          n277 = call "IMAQ AVI Close"("error in (no error)"=w186, "Avi Refnum"=w184) -> ("error out"=w185:errorcluster)  [unwired: 9 out]
          n278 = Release Queue(queue=w189, error in (no error)=w185) -> (error out=w175:errorcluster)  [unwired: 1 in, 2 out]
          n279 = Close File(refnum=w176, error in=w177) -> ()  [unwired: 2 out]
          n280 = call <vilib>:"Simple Error Handler.vi"("error in (no error)"=w175) -> ()  [unwired: 4 in, 5 out]
          n281 = Request Deallocation(TRUE ("flag")) -> ()
          n282 = call <vilib>:"Simple Error Handler.vi"("error in (no error)"=w168) -> ()  [unwired: 4 in, 5 out]
          n283 = call <vilib>:"IMAQdx Close Camera.vi"("error in"=w200, "Session In"=w199) -> ("error out"=w198:errorcluster)  [unwired: 9 in]
          n284 = call "IMAQ Dispose"("error in (no error)"=w198) -> ("error out"=w197:errorcluster)  [unwired: 5 in]
          n285 = call <vilib>:"Simple Error Handler.vi"("error in (no error)"=w197) -> ()  [unwired: 4 in, 5 out]
        }
        frame #1 {
          w424 = u8 1 ("Response to Value Outside Limits:Minimum")
          # "Stop an acquisition if still running"
          n286 = property on="imageNo" class="DigNum (strict)"("OutOfRngActMin"=w424) -> ()  [unwired: 2 in, 2 out]
          n287 = property on="imageNo" class="DigNum (strict)"("OutOfRngActMax"=w424) -> ()  [unwired: 2 in, 2 out]
          n288 = local read "Handle"() -> (w426:i32)
          n289 = property on="imageNo" class="DigNum (strict)"("Minimum"=w424) -> ()  [unwired: 2 in, 2 out]
          n290 = call <userlib>:"AT Command A.vi"("Feature"="AcquisitionStop" ("Command"), "Handle"=w426) -> ()  [unwired: 8 in, 2 out]
        }
      }
    }
    frame #11 {
      # "Create an event handler so that when the user selects a frame the display is updated"
      n291 = stacked-sequence {
        frame #0 {
          w427 = T4."Enabled" ("Disabled")
          n292 = property on="imageNo" class="DigNum (strict)"("DisabledEnum"=w427) -> ()  [unwired: 2 in, 2 out]
          n293 = property on="stop" class="Bool (strict)"("DisabledEnum"=w427) -> ()  [unwired: 2 in, 2 out]
        }
        frame #1 {
          n294 = while {
            stop <- w428 stop-if-true
            n295 = event shown="[0] Timeout" {
              selector: _ -> [_ _]
              dyn-events: _ -> [_ _]
              timeout: 100 -> [_ _]
              event Timeout {
                n296 = event-data() -> ()  [unwired: 1 in, 2 out]
              }
              event "imageNo": Value Change {
                # "Display the currently selected frame"
                n297 = event-data() -> ()  [unwired: 1 in, 5 out]
                n298 = local read "image pointers"() -> (w441:u64[])
                n299 = local read "imageNo"() -> (w435:i32)
                n300 = Decrement(x=w435) -> (x-1=w436:i32)
                n301 = local read "ImageSizeBytes"() -> (w434:i64)
                n302 = local read "ByteData"() -> (w433:u8[])
                n303 = Index Array(array=w441, index=w436) -> (element=w432:u64)
                n304 = local read "Pixel Encoding"() -> (w443:string)
                n305 = local read "AOI Height"() -> (w439:i64)
                n306 = local read "AOIStride"() -> (w442:i64)
                n307 = local read "AOI Width"() -> (w438:i64)
                n308 = local read "PixelData"() -> (w444:u16[])
                n309 = call <userlib>:"PointerToArrayEX.vi"("Array in"=w433, "Pointer In"=w432, "Pointer Size"=w434) -> ("Array out"=w431:u8[], "error out"=w430:errorcluster)  [unwired: 5 in]
                n310 = call-poly <userlib>:"GetPixelData.vi"("Input buffer"=w431, "Output buffer in"=w444, "Pixel Encoding"=w443, "Stride"=w442, "error in (no error)"=w430, "Width"=w438, "Height"=w439) -> ("Output buffer out"=w440:u16[])  [unwired: 10 in, 2 out]
                n311 = Reshape Array(w440, w439, w438) -> (w437:u16[][])
                n312 = local write "Intensity Graph"(w437) -> ()
              }
            }
            n313 = local read "stop"() -> (w428:bool)
          }
        }
      }
    }
    frame #12 {
      w445 = T4."Enabled" ("Disabled")
      # "re-enable controls"
      n314 = property on="AOI Height" class="DigNum (strict)"("DisabledEnum"=w445) -> ()  [unwired: 2 in, 2 out]
      n315 = property on="AOI Width" class="DigNum (strict)"("DisabledEnum"=w445) -> ()  [unwired: 2 in, 2 out]
      n316 = property on="PreAmp Gain Control" class="CmbBox"("DisabledEnum"=w445) -> ()  [unwired: 2 in, 2 out]
      n317 = property on="Centre AOI" class="Bool (strict)"("DisabledEnum"=w445) -> ()  [unwired: 2 in, 2 out]
      n318 = property on="NumImages" class="DigNum (strict)"("DisabledEnum"=w445) -> ()  [unwired: 2 in, 2 out]
    }
    frame #13 {
      # "Close the current camera handle and unload the library"
      # "ShutDown."
      n319 = local write "Ready"(FALSE ("Ready")) -> ()
      n320 = local read "Handle"() -> (w447:i32)
      n321 = call <userlib>:"AT Clear All Buffers A.vi"("Handle"=w447) -> ("error out"=w446:errorcluster)  [unwired: 9 in, 1 out]
      n322 = call <userlib>:"AT Close A.vi"("error in (no error)"=w446, "Handle"=w447) -> ("error out"=w448:errorcluster)  [unwired: 8 in, 1 out]
      n323 = call <userlib>:"AT Finalise Library A.vi"("error in (no error)"=w448) -> ()  [unwired: 9 in, 2 out]
    }
  }
  "Ready" <- FALSE ("Ready")
